vi "Catagoried alarms combine.vi"(5 "Catagorised  Stsaus 1":T1[](array[typedef]), 7 "Catagorised  Stsaus 2":T1[](array[typedef]), 9 "Catagorised  Stsaus 3":T1[](array[typedef]), 11 "Catagorised  Stsaus 4":T1[](array[typedef])) -> (6 "catagorised Status out":T1[](array[typedef]), 10 "Catagoried alarms out":bool[](array[boolean]))   [LabVIEW 2011]
uses:
  Catagorised alarm state.ctl
  GUI/Status Indikator Helper.ctl
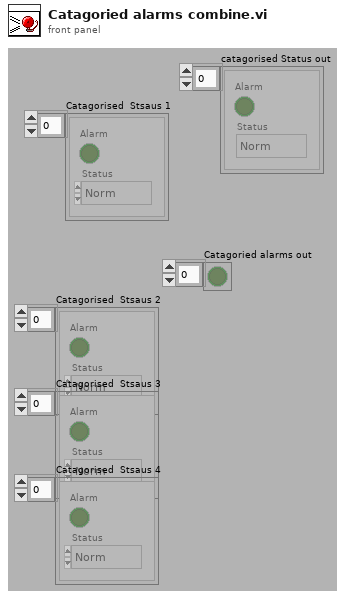
[diagram p1: front panel]
types:
  T1 = typedef "Catagorised alarm state.ctl" = cluster{"Alarm":bool, "Status":T2}
  T2 = typedef "Status Indikator Helper.ctl" = enum16{"Norm", "L", "H", "LL", "HH", "Value", "Technical"}
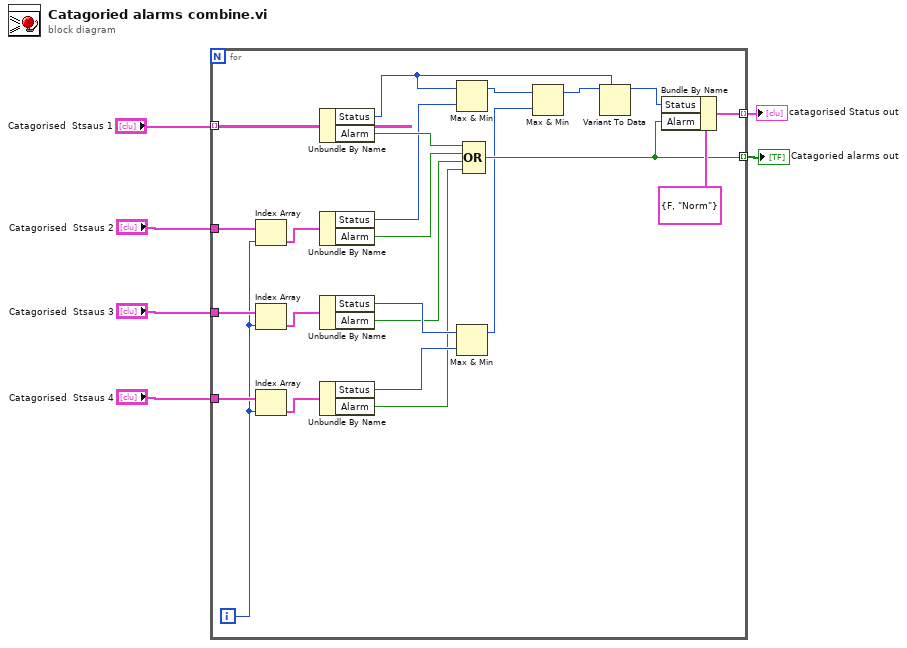
[diagram p0: block diagram]
diagram:
  n1 = for {
    tunnel: [w23] -> w6 mode=indexing
    tunnel: "Catagorised  Stsaus 1" -> [w29] mode=indexing
    tunnel: "Catagorised  Stsaus 2" -> [w20]
    tunnel: [w21] -> w3 mode=indexing
    tunnel: "Catagorised  Stsaus 3" -> [w17]
    tunnel: "Catagorised  Stsaus 4" -> [w16]
    i -> [w14]
    n2 = Index Array(array=w20, index=w14) -> (element=w19:T1)
    n3 = Index Array(array=w17, index=w14) -> (element=w18:T1)
    n4 = Index Array(array=w16, index=w14) -> (element=w15:T1)
    n5 = Unbundle By Name(w29) -> ("Status"=w28:T2, "Alarm"=w27:bool)
    n6 = Unbundle By Name(w19) -> ("Status"=w26:T2, "Alarm"=w25:bool)
    n7 = Unbundle By Name(w18) -> ("Status"=w12:T2, "Alarm"=w8:bool)
    n8 = Unbundle By Name(w15) -> ("Status"=w11:T2, "Alarm"=w7:bool)
    n9 = Max & Min(x=w28, y=w26) -> (max(x,y)=w13:u16)  [unwired: 1 out]
    n10 = Max & Min(x=w12, y=w11) -> (max(x,y)=w10:u16)  [unwired: 1 out]
    n11 = Compound Arithmetic op=OR(w27, w25, w8, w7) -> (w23:bool)
    n12 = Max & Min(x=w13, y=w10) -> (max(x,y)=w9:u16)  [unwired: 1 out]
    n13 = Variant To Data(type=w28, Variant=w9) -> (data=w22:T2)  [unwired: 1 in, 1 out]
    n14 = Bundle By Name(cluster=T1 {"Alarm"=FALSE, "Status"=enum."Norm"} ("catagori"), "Status"=w22, "Alarm"=w23) -> (w21:T1)
  }
  "Catagoried alarms out" <- w6
  "catagorised Status out" <- w3
